vi "RTG_QMH_Main.vi"() -> ()   [LabVIEW 2020]
uses:
  <vilib>/RTG/API/interface/public/State.ctl
  <vilib>/RTG/API/ip/common/host-types/Target Configuration.ctl
  <vilib>/RTG/API/ip/common/host-types/Synchronization - Host.ctl
  <vilib>/RTG/API/ip/common/host-types/Synchronization Mode - Host.ctl
  <vilib>/RTG/API/ip/common/host-types/Basic Target - Host.ctl
  <vilib>/RTG/API/ip/common/host-types/Target Motion Parameters.ctl
  <vilib>/RTG/API/ip/common/host-types/Single Target Motion Parameters.ctl
  <vilib>/RTG/API/interface/public/Coprocessor Link Status.ctl
  <vilib>/RTG/coprocessor/host/RTG Coprocessor Link Interface/Public/Coprocessor Status.ctl
  Controls/Enum/Program_Status_Enum.ctl
  Controls/Enum/Supervisor_Enum.ctl
  Controls/Enum/RTG_Enum.ctl
  Controls/Clust/RTG Clust.ctl
  <vilib>/RTG/API/interface/NI-RTG Interface.lvclass
  Controls/Clust/CoProcessor Clust.ctl
  <vilib>/RTG/coprocessor/host/RTG Coprocessor Link Interface/RTG Coprocessor Link Interface.lvclass
  Controls/Enum/CoProcessor_Enum.ctl
  Controls/Clust/RTG API Clust.ctl
  support/Options - API Mode.ctl
  support/Options - Calibration.ctl
  support/Options - Remote.ctl
  <vilib>/Utility/error.llb/Error Cluster From Error Code.vi
  <vilib>/rvi/errors/niLvFpgaAdjustHostInterfaceError.vi
  <vilib>/rvi/interface/nirviReadWriteControl/nirviReadWriteControl.xnode
  RTG Examples.lvlib
  <vilib>/RTG/API/ip/common/host-types/Host Data Types v1.lvlib
  NiFpgaLv.dll
  <vilib>/rvi/interface/Simulation/niFpgaSimulationCallBeginRW.vi
panel:
  out "App Status":T1
  in  "Tab Control":T2(tab)
  in  "Instrument Names":string[](array[string])=["5831_0"]
  in  "Coprocessor Names":string[](array[string])
  in  "Center Freqeuncies (Hz)":dbl[](array[numeric])=[5500000000.0] format="%#_6p"
  in  "Reference Levels (dBm)":dbl[](array[numeric])=[0.0]
  in  "Calibrate":bool=TRUE
  in  "abort system self cal":bool
  in  "Commit HW":bool
  in  "ExtAtten":dbl[](array[numeric]) caption="External Attenuations (dB)"
  in  "OffsFreq":dbl[](array[numeric]) caption="Offset Frequencies (Hz)" format="%#_6p"
  in  "ExtDelay":dbl[](array[numeric]) caption="External Delay (s)" format="%#_6p"
  in  "mmWave Radio Heads Enable":bool[](array[boolean])
  in  "PRI (s)":dbl[](array[numeric]) format="%#_6p"
  in  "Set PRIs":bool
  out "Min Latencies (s)":dbl[](array[numeric]) format="%#_6p"
  out "Min Common Attenuations (dB)":dbl[](array[numeric])
  out "Max Common Attenuations (dB)":dbl[](array[numeric])
  out "Versions":string[](array[string])
  in  "Common Attenuation (dB)":dbl
  in  "Auto Send Software Trigger":bool
  in  "Prepend Software Trigger":bool
  in  "Device Index":i32
  in  "Target Configuration Files":path[](array[path])
  in  "Target Configuration":T3 {"rtg targets"."time offset (s)" format="%#_6p"; "rtg targets"."doppler" format="%#_6p"}
  in  "Target Motion Parameters":T7={"target motions"=[{"target enable"=FALSE, "start time offset (s)"=-1e-09, "time offset rate of change (s/s)"=0.001, "start attenuation (dB)"=0.0, "attenuation rate of change (dB/s)"=0.0, "start frequency shift (Hz)"=0.0, "frequency shift rate of change (Hz/sec)"=0.0}], "scenario duration (s)"=67.0, "configuration update rate(Hz)"=15000.0} {"configuration update rate(Hz)" format="%#_6p"; "target motions"."frequency shift rate of change (Hz/sec)" format="%#_6p"; "target motions"."start frequency shift (Hz)" format="%#_6p"; "target motions"."time offset rate of change (s/s)" format="%#_6p"; "target motions"."start time offset (s)" format="%#_6p"}
  in  "Send TrgtCfg":bool
  in  "Send Motion":bool
  in  "Send Files":bool
  in  "Start RTG":bool
  in  "Stop RTG":bool
  in  "Send SW Trigg":bool
  out "rtg link status":T9[](array[typedef])
  out "Trigger Count":i32[][](array[numeric]) caption="Device Index vs Trigger Count"
  out "RTG Status":string
  out "RTG State":T10
  out "error out":errorcluster
  out "System Time":string
  out "coproc link":T11[](array[typedef]) caption="coprocessor link status"
  in  "Exit":bool
  # "v20230906"
  # "Configuration Files and Target Motion"
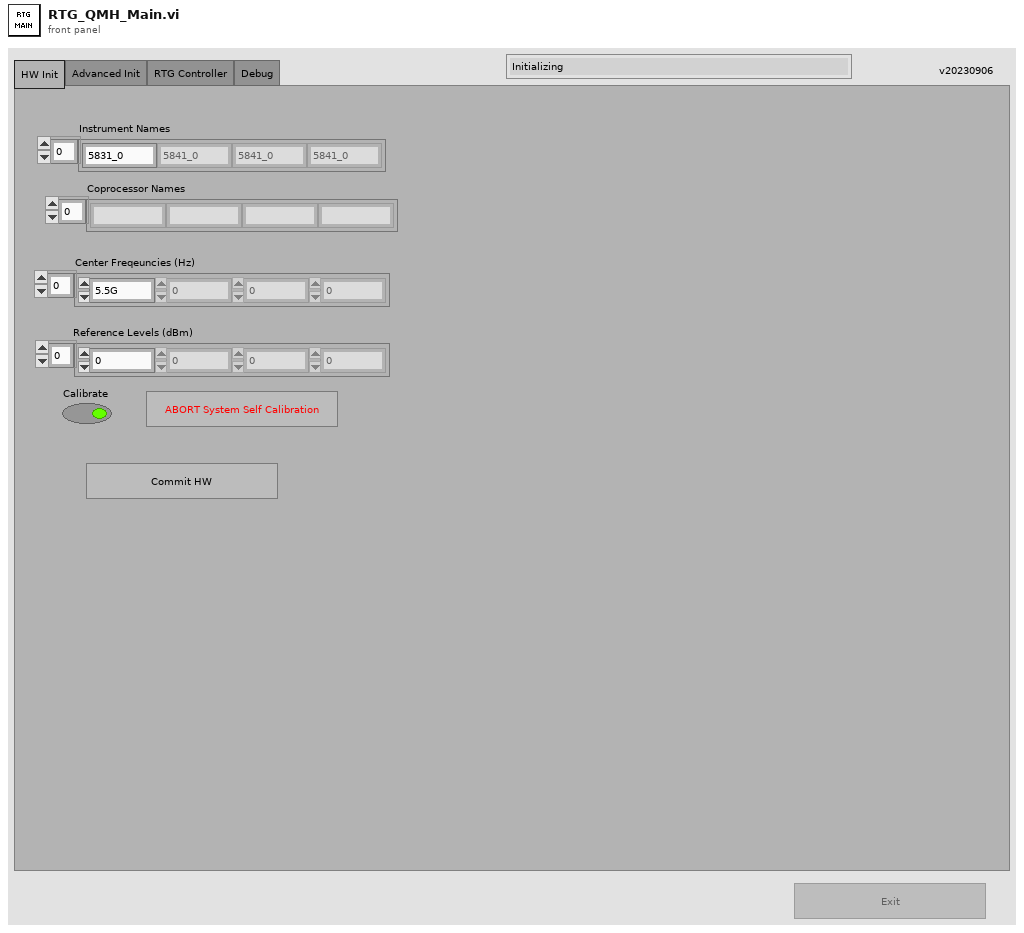
[diagram p1: front panel]
types:
  T1 = typedef "Program_Status_Enum.ctl" = enum16{"Initializing", "RTG Inactive", "Unconfigured", "RTG active", "Error", "Closing", "Closed"}
  T2 = enum32{"HW Init", "Advanced Init", "RTG Controller", "Debug"}
  T3 = typedef "Host Data Types v1.lvlib/Target Configuration.ctl" = cluster{"synchronization":T4, "rtg targets":T6[]}
  T4 = typedef "Host Data Types v1.lvlib/Synchronization - Host.ctl" = cluster{"synch mode":T5, "time offset (s)":dbl}
  T5 = typedef "Host Data Types v1.lvlib/Synchronization Mode - Host.ctl" = enum16{"Software Trigger", "Hardware Trigger", "Time Offset Relative to First", "Time Offset Relative to Last", "Pulse Rising Edge", "Pulse Falling Edge"}
  T6 = typedef "Host Data Types v1.lvlib/Basic Target - Host.ctl" = cluster{"time offset (s)":dbl, "attenuaton (dB)":dbl, "doppler":dbl, "target enable":bool, "relative velocity enable":bool}
  T7 = typedef "Host Data Types v1.lvlib/Target Motion Parameters.ctl" = cluster{"target motions":T8[], "scenario duration (s)":dbl, "configuration update rate(Hz)":dbl}
  T8 = typedef "Host Data Types v1.lvlib/Single Target Motion Parameters.ctl" = cluster{"target enable":bool, "start time offset (s)":dbl, "time offset rate of change (s/s)":dbl, "start attenuation (dB)":dbl, "attenuation rate of change (dB/s)":dbl, "start frequency shift (Hz)":dbl, "frequency shift rate of change (Hz/sec)":dbl}
  T9 = typedef "NI-RTG v1.lvlib/NI-RTG Interface.lvclass/Coprocessor Link Status.ctl" = cluster{"task name":string, "device name":string, "hard error":bool, "soft error":bool, "channel up":bool, "system reset":bool}
  T10 = typedef "NI-RTG v1.lvlib/NI-RTG Interface.lvclass/State.ctl" = enum16{"Idle", "Inactive", "Active", "System Self Calibration"}
  T11 = typedef "RTG Coprocessor Link Interface v1 Host.lvlib/RTG Coprocessor Link Interface.lvclass/Coprocessor Status.ctl" = cluster{"tx read count":u64, "tx read overflow":bool, "rx read count":u64, "rx read overflow":bool}
  T12 = typedef "CoProcessor_Enum.ctl" = enum16{"CoPr_Init", "CoPr_Chk", "CoPr_Exit"}
  T13 = typedef "CoProcessor Clust.ctl" = cluster{"CoPr Refs":refnum<class "RTG Coprocessor Link Interface.lvclass">[]}
  T14 = typedef "RTG Clust.ctl" = cluster{"VST_Names":string[], "OptionString":string, "RTG Ref":refnum<class "NI-RTG Interface.lvclass">, "Index":i32, "AutoSend":bool, "Prepend":bool, "state":T10}
  T15 = typedef "RTG_Enum.ctl" = enum16{"RTG_InitHW", "RTG_RefLvl", "RTG_mmWav", "RTG_Cal", "RTG_CalDone?", "RTG_ExtAtten", "RTG_GetCal", "RTG_SetPRIs", "RTG_CommAtten", "RTG_TargetSetup", "RTG_Send Files", "RTG_Send Target Cfg", "RTG_Send Motion", "RTG_Send SW Trigg", "RTG_Start", "RTG_Stop", "RTG_Chk", "RTG_Exit"}
  T16 = typedef "Supervisor_Enum.ctl" = enum16{"Spvsr_InitSW", "Spvsr_InitCtrls", "Spvsr_UpdtFP", "Spvsr_InitRTG", "Spvsr_StateCount", "Spvsr_Exit"}
  T17 = enum8{"Enabled", "Disabled", "Disabled and Grayed Out"}
  T18 = typedef "RTG API Clust.ctl" = cluster{"Local?":T19, "Cal":T20, "Remote":T21, "ini path":path}
  T19 = typedef "RTG Examples.lvlib/Options - API Mode.ctl" = enum16{"Local", "Remote"}
  T20 = typedef "RTG Examples.lvlib/Options - Calibration.ctl" = cluster{"enable internal loopback  ":bool, "enable overwrite cal data  ":bool, "enable save cal data           ":bool, "disable self cal range          ":bool}
  T21 = typedef "RTG Examples.lvlib/Options - Remote.ctl" = cluster{"ip address":string, "port":string, "certificate path":path, "timeout (ms)":i32}
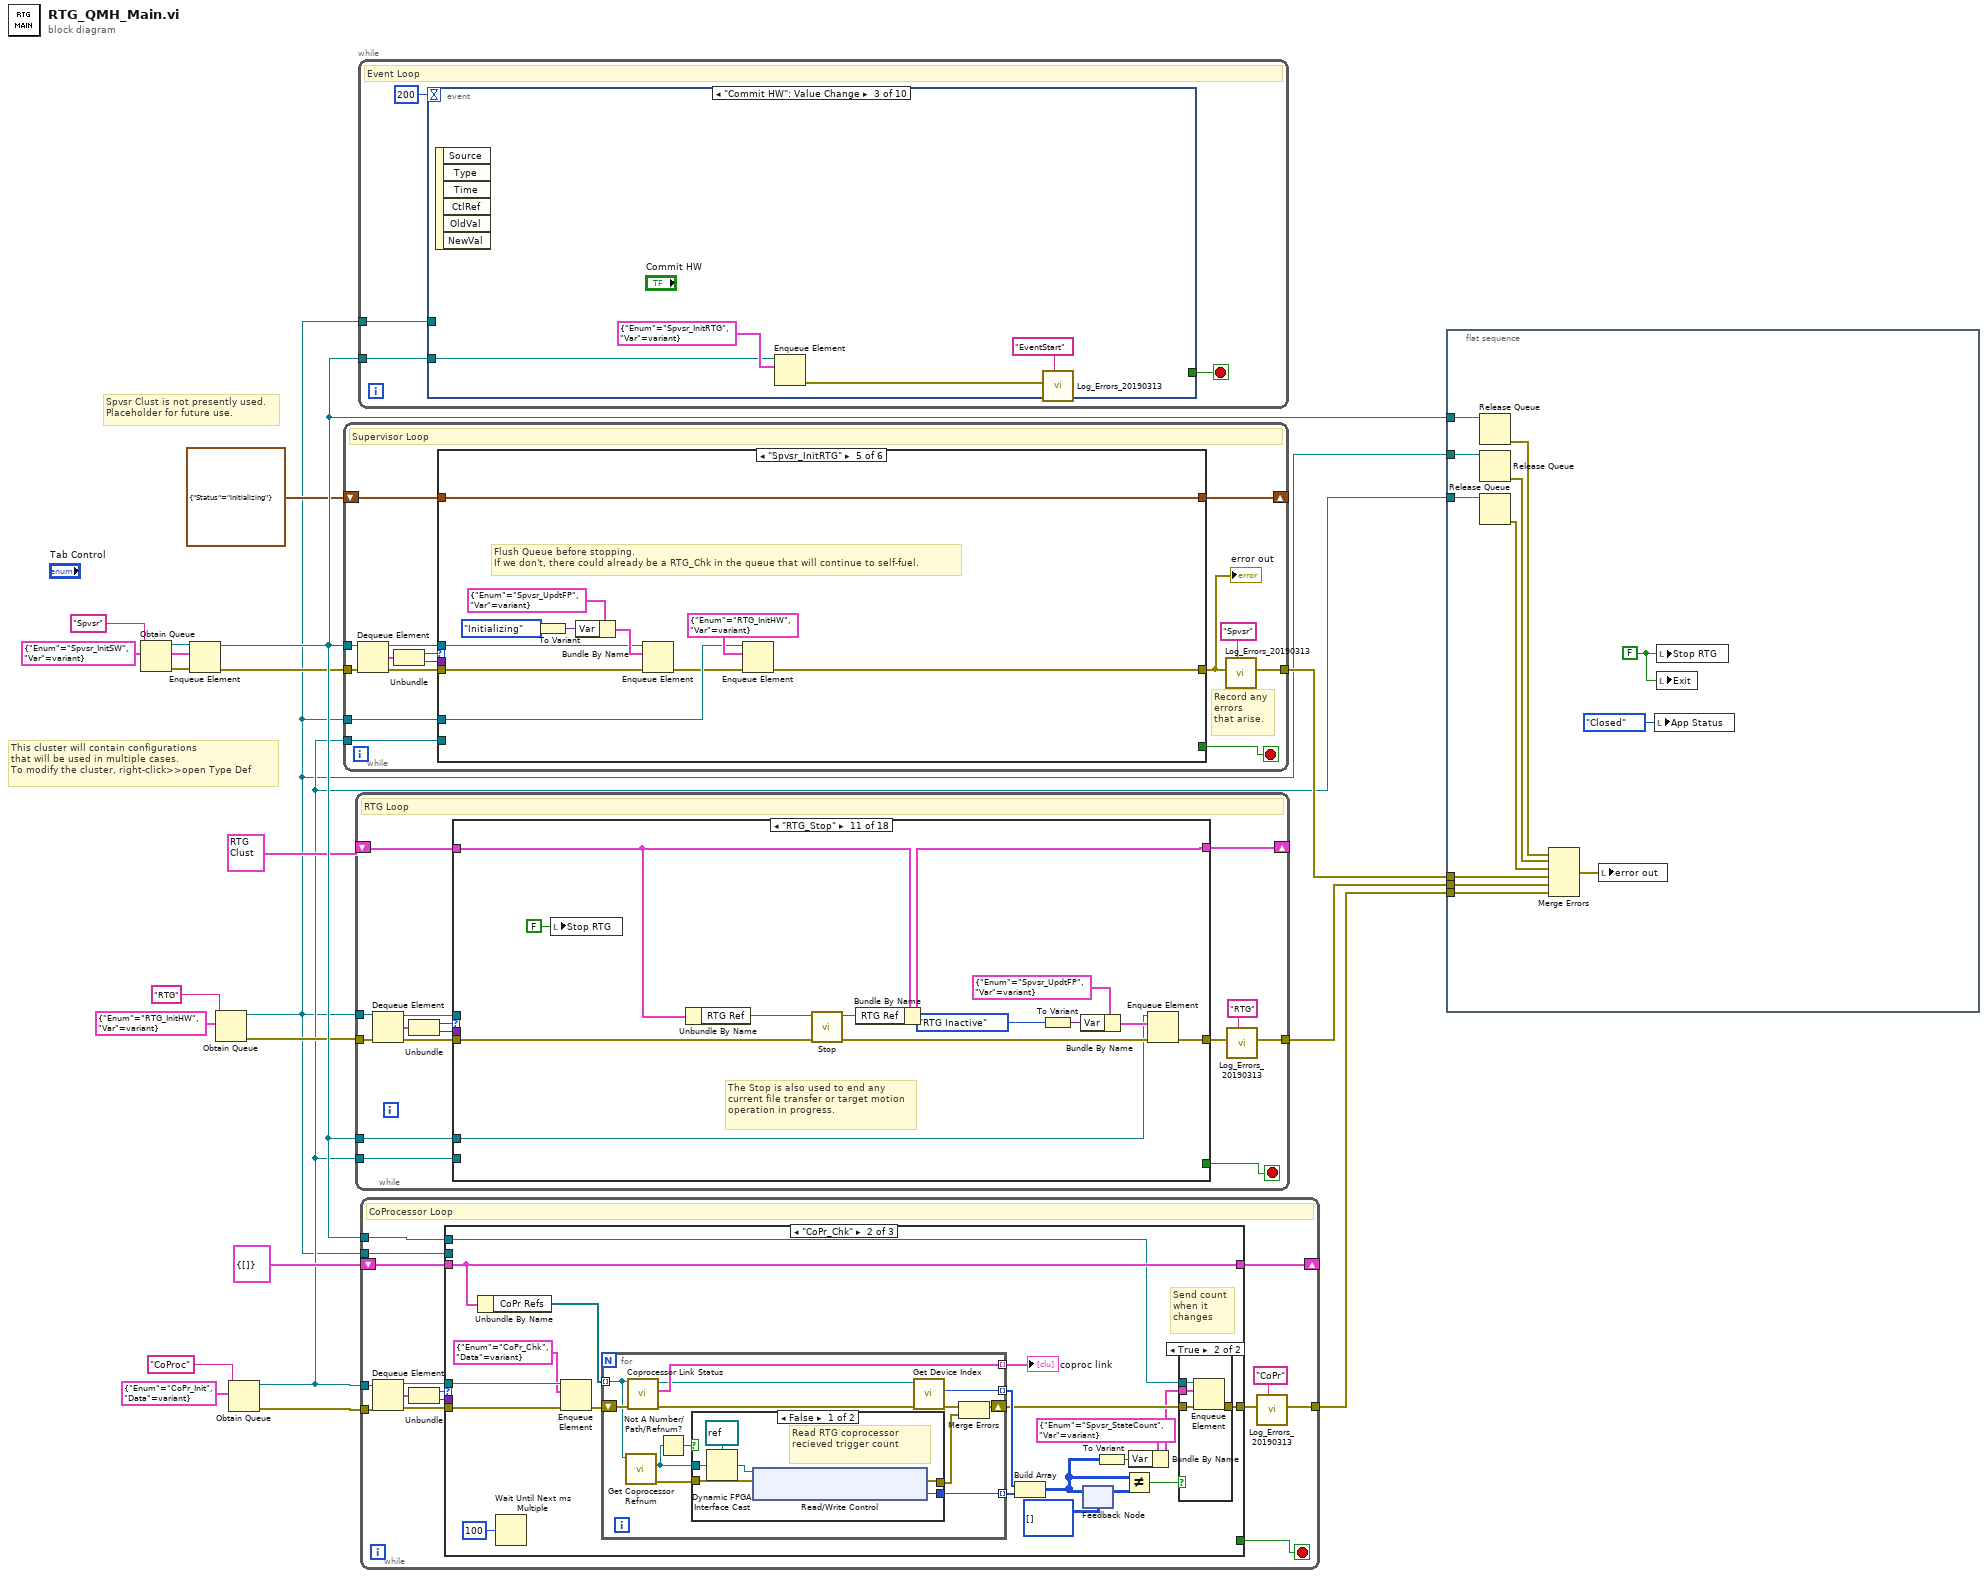
[diagram p0: block diagram]
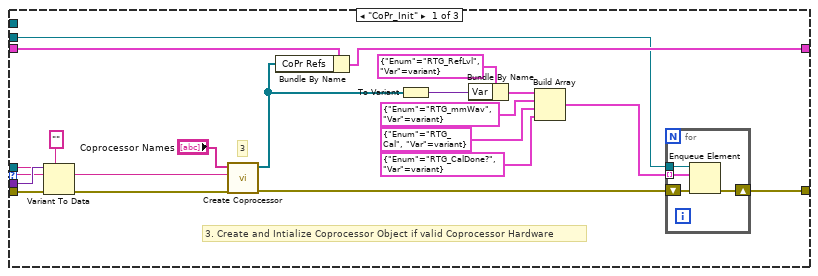
[diagram p2: hidden frame]
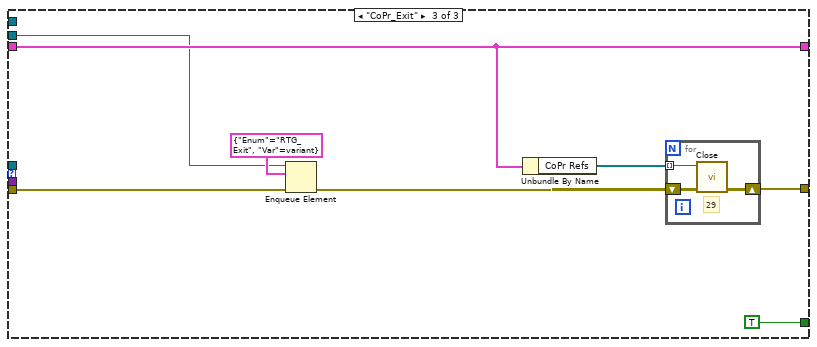
[diagram p5: hidden frame]
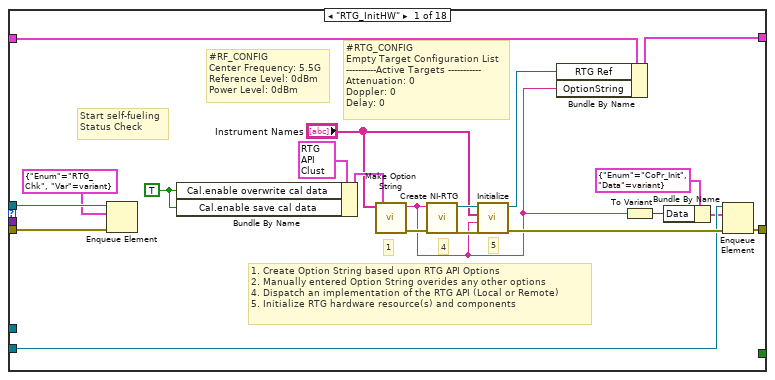
[diagram p6: hidden frame]
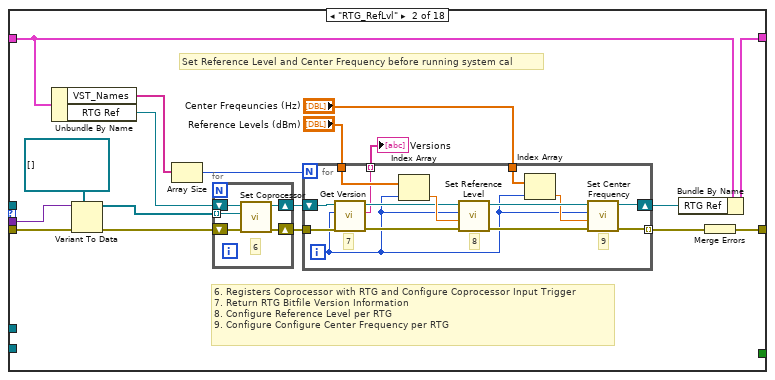
[diagram p7: hidden frame]
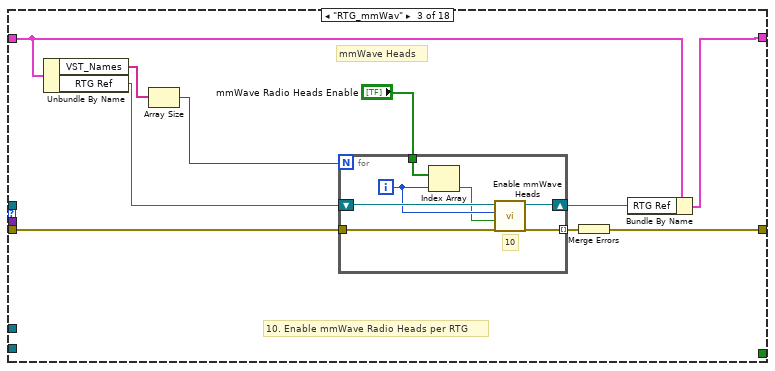
[diagram p8: hidden frame]
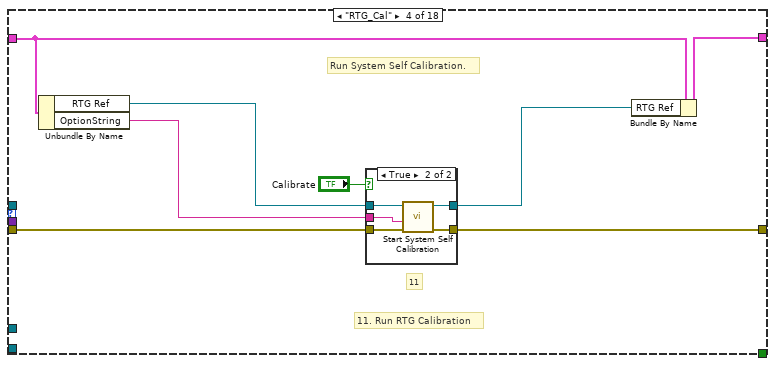
[diagram p9: hidden frame]
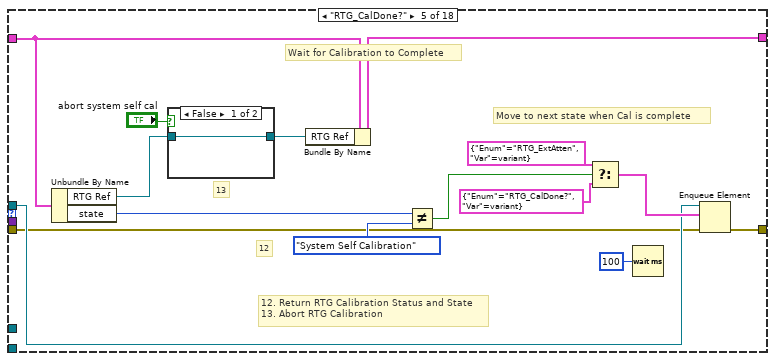
[diagram p11: hidden frame]
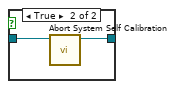
[diagram p12: hidden frame]
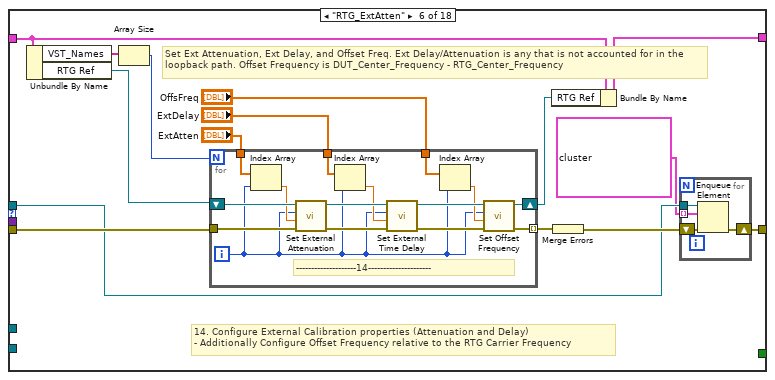
[diagram p13: hidden frame]
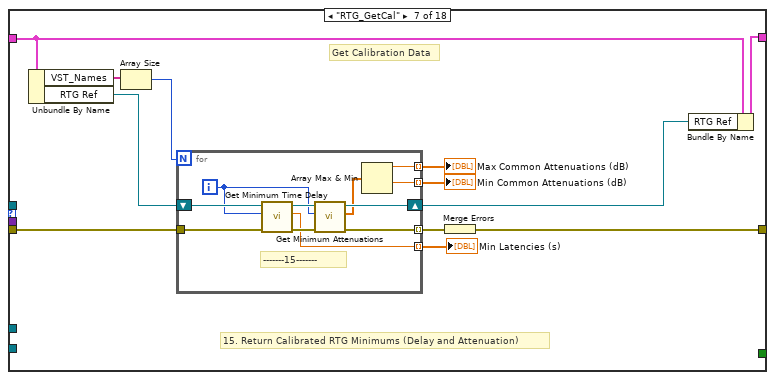
[diagram p14: hidden frame]
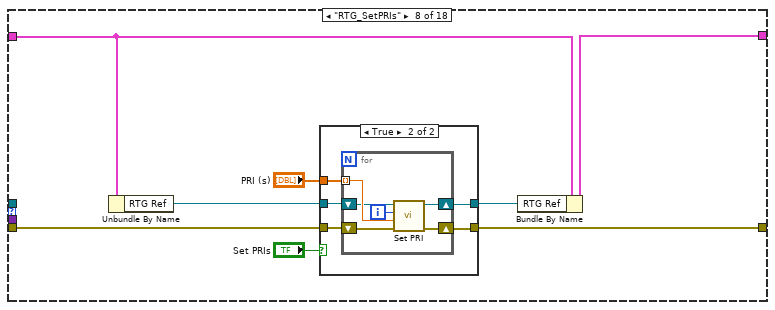
[diagram p15: hidden frame]
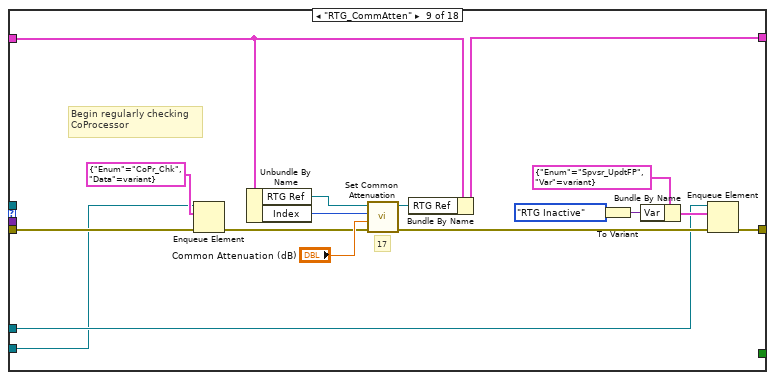
[diagram p17: hidden frame]
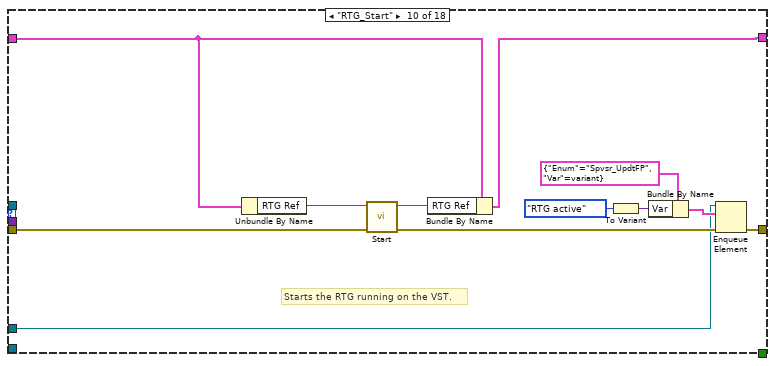
[diagram p18: hidden frame]
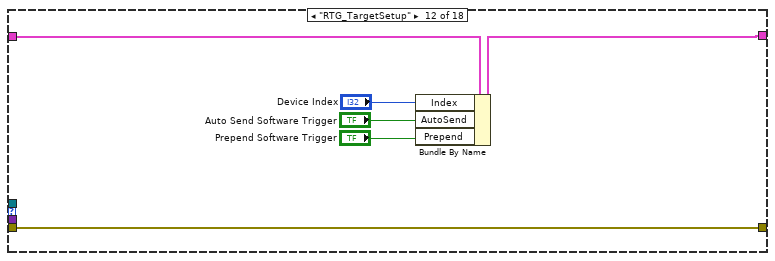
[diagram p19: hidden frame]
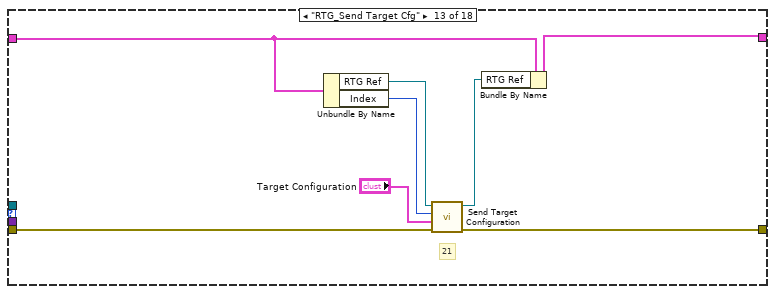
[diagram p20: hidden frame]
diagram:
  w16 = cluster{"Enum":T16, "Var":variant} {"Enum"=enum."Spvsr_InitSW", "Var"=variant}
  # "Spvsr Clust is not presently used.\nPlaceholder for future use."
  # "This cluster will contain configurations\nthat will be used in multiple cases.\nTo modify the cluster, right-click>>open Type Def"
  n1 = Obtain Queue(name (unnamed)="Spvsr", element data type=w16) -> (queue out=w17:refnum<queue>, error out=w19:errorcluster)  [unwired: 3 in, 1 out]
  n2 = Enqueue Element(queue=w17, element=w16, error in (no error)=w19) -> (queue out=w20:refnum<queue>, error out=w18:errorcluster)  [unwired: 1 in, 1 out]
  n3 = Obtain Queue(name (unnamed)="RTG", element data type=cluster{"Enum":T15, "Var":variant} {"Enum"=enum."RTG_InitHW", "Var"=variant}) -> (queue out=w1:refnum<queue>, error out=w14:errorcluster)  [unwired: 3 in, 1 out]
  n4 = Obtain Queue(name (unnamed)="CoProc", element data type=cluster{"Enum":T12, "Data":variant} {"Enum"=enum."CoPr_Init", "Data"=variant}) -> (queue out=w2:refnum<queue>, error out=w12:errorcluster)  [unwired: 3 in, 1 out]
  n5 = while {
    tunnel: w18 -> [w35]
    tunnel: w20 -> [w33]
    tunnel: w1 -> [w28]
    tunnel: [w25] -> w6
    tunnel: w2 -> [w24]
    shift-right: [w22] -> _
    shift-left: cluster{"Status":T1} {"Status"=enum."Initializing"} -> [w23]
    stop <- w21 stop-if-true
    # "Record any\nerrors \nthat arise."
    # "Supervisor Loop"
    n6 = Dequeue Element(queue=w33, error in (no error)=w35) -> (queue out=w31:refnum<queue>, element=w32:cluster{"Enum":T16, "Var":variant}, error out=w34:errorcluster)  [unwired: 1 in, 1 out]
    n7 = Unbundle(w32) -> ("Enum"=w30:T16, "Var"=w29:variant)
    n8 = case shown="\"Spvsr_InitRTG\"" w30 {
      tunnel: w34 -> [w46 w48 w59 w121 w127 w139]
      tunnel: w31 -> [w45 w47 _ _ w124 _]
      tunnel: w29 -> [_ _ w58 _ _ w137]
      tunnel: w28 -> [_ _ _ w119 w133 _]
      tunnel: [w43 w49 w61 w118 w125 w135] -> w26
      tunnel: w24 -> [_ _ _ w116 _ _]
      tunnel: w23 -> [w36 w54 w74 w112 w132 w140]
      tunnel: [w36 w54 w74 w112 w132 w140] -> w22
      tunnel: [_ _ _ TRUE _ _] -> w21
      frame "Spvsr_InitSW" {
        n9 = Enqueue Element(queue=w45, element=cluster{"Enum":T16, "Var":variant} {"Enum"=enum."Spvsr_InitCtrls", "Var"=variant}, error in (no error)=w46) -> (queue out=w41:refnum<queue>, error out=w42:errorcluster)  [unwired: 1 in, 1 out]
        n10 = To Variant(anything=Program_Status_Enum."Initializing" ("Status")) -> (Variant=w38:variant)
        n11 = Bundle By Name(cluster=cluster{"Enum":T16, "Var":variant} {"Enum"=enum."Spvsr_UpdtFP", "Var"=variant}, "Var"=w38) -> (w37:cluster{"Enum":T16, "Var":variant})
        n12 = Enqueue Element(queue=w41, element=w37, error in (no error)=w42) -> (error out=w43:errorcluster)  [unwired: 1 in, 2 out]
      }
      frame "Spvsr_InitCtrls" {
        w55 = FALSE ("Exit")
        n13 = To Variant(anything=Program_Status_Enum."Unconfigured" ("Status")) -> (Variant=w53:variant)
        n14 = Bundle By Name(cluster=cluster{"Enum":T16, "Var":variant} {"Enum"=enum."Spvsr_UpdtFP", "Var"=variant}, "Var"=w53) -> (w51:cluster{"Enum":T16, "Var":variant})
        n15 = Enqueue Element(queue=w47, element=w51, error in (no error)=w48) -> (error out=w49:errorcluster)  [unwired: 1 in, 2 out]
        n16 = local write "Exit"(w55) -> ()
        n17 = local write "Stop RTG"(w55) -> ()
      }
      frame "Spvsr_UpdtFP" {
        n18 = Variant To Data(error in=w59, type=Program_Status_Enum."Closed" ("App Status"), Variant=w58) -> (data=w56:T1, error out=w60:errorcluster)
        "App Status" <- w56
        n19 = case shown="\"Unconfigured\"" w56 {
          tunnel: [T17."Disabled and Grayed Out" ("Disabled") T17."Enabled" ("Disabled") T17."Disabled and Grayed Out" ("Disabled") T17."Disabled and Grayed Out" ("Disabled") T17."Enabled" ("Disabled") T17."Disabled and Grayed Out" ("Disabled")] -> w67
          tunnel: [T17."Disabled and Grayed Out" ("Disabled") T17."Enabled" ("Disabled") T17."Disabled and Grayed Out" ("Disabled") T17."Disabled and Grayed Out" ("Disabled") T17."Disabled and Grayed Out" ("Disabled") T17."Enabled" ("Disabled")] -> w66
          tunnel: [T17."Enabled" ("Disabled") T17."Enabled" ("Disabled") T17."Disabled and Grayed Out" ("Disabled") T17."Enabled" ("Disabled") T17."Enabled" ("Disabled") T17."Enabled" ("Disabled")] -> w65
          tunnel: [T17."Disabled and Grayed Out" ("Disabled") T17."Disabled and Grayed Out" ("Disabled") T17."Disabled and Grayed Out" ("Disabled") T17."Disabled and Grayed Out" ("Disabled") T17."Disabled and Grayed Out" ("Disabled") T17."Enabled" ("Disabled")] -> w64
          tunnel: [T17."Disabled and Grayed Out" ("Disabled") T17."Disabled and Grayed Out" ("Disabled") T17."Disabled and Grayed Out" ("Disabled") T17."Disabled and Grayed Out" ("Disabled") T17."Disabled and Grayed Out" ("Disabled") T17."Enabled" ("Disabled")] -> w63
          tunnel: [T17."Disabled and Grayed Out" ("Disabled") T17."Disabled and Grayed Out" ("Disabled") T17."Disabled and Grayed Out" ("Disabled") T17."Disabled and Grayed Out" ("Disabled") T17."Disabled and Grayed Out" ("Disabled") T17."Enabled" ("Disabled")] -> w62
          frame "Unconfigured" {
          }
          frame "Error" {
          }
          frame "Closing", "Closed" {
          }
          frame "Initializing" {
          }
          frame "RTG Inactive" {
          }
          frame "RTG active" {
          }
        }
        n20 = property on="Start RTG" class="Bool"(error in=w60, "DisabledEnum"=w67) -> (error out=w68:errorcluster)  [unwired: 1 in, 1 out]
        n21 = property on="Stop RTG" class="Bool (strict)"("DisabledEnum"=w66) -> (error out=w69:errorcluster)  [unwired: 2 in, 1 out]
        n22 = property on="Exit" class="Bool (strict)"("DisabledEnum"=w65) -> (error out=w70:errorcluster)  [unwired: 2 in, 1 out]
        n23 = property on="Send TrgtCfg" class="Bool"("DisabledEnum"=w64) -> (error out=w71:errorcluster)  [unwired: 2 in, 1 out]
        n24 = property on="Send Motion" class="Bool"("DisabledEnum"=w63) -> (error out=w72:errorcluster)  [unwired: 2 in, 1 out]
        n25 = property on="Send Files" class="Bool"("DisabledEnum"=w62) -> (error out=w73:errorcluster)  [unwired: 2 in, 1 out]
        n26 = Merge Errors(w68, w69, w70, w71, w72, w73) -> (w61:errorcluster)
      }
      frame "Spvsr_Exit" {
        # "RTG Exit is called from Coprocesor Exit\nto prevent a race condition"
        # "Flush Queue before stopping.\nIf we don't, there could already be a RTG_Chk in the queue that will continue to self-fuel."
        n27 = Flush Queue(queue=w119, error in (no error)=w121) -> (queue out=w120:refnum<queue>, error out=w122:errorcluster)  [unwired: 1 out]
        n28 = Enqueue Element(queue=w120, element=cluster{"Enum":T15, "Var":variant} {"Enum"=enum."RTG_Stop", "Var"=variant}, error in (no error)=w122) -> (error out=w114:errorcluster)  [unwired: 1 in, 2 out]
        n29 = Flush Queue(queue=w116, error in (no error)=w114) -> (queue out=w115:refnum<queue>, error out=w113:errorcluster)  [unwired: 1 out]
        n30 = Enqueue Element(queue=w115, element=cluster{"Enum":T12, "Data":variant} {"Enum"=enum."CoPr_Exit", "Data"=variant}, error in (no error)=w113) -> (error out=w118:errorcluster)  [unwired: 1 in, 2 out]
      }
      frame "Spvsr_InitRTG" {
        # "Flush Queue before stopping.\nIf we don't, there could already be a RTG_Chk in the queue that will continue to self-fuel."
        n31 = To Variant(anything=Program_Status_Enum."Initializing" ("Status")) -> (Variant=w131:variant)
        n32 = Bundle By Name(cluster=cluster{"Enum":T16, "Var":variant} {"Enum"=enum."Spvsr_UpdtFP", "Var"=variant}, "Var"=w131) -> (w129:cluster{"Enum":T16, "Var":variant})
        n33 = Enqueue Element(queue=w124, element=w129, error in (no error)=w127) -> (error out=w126:errorcluster)  [unwired: 1 in, 2 out]
        n34 = Enqueue Element(queue=w133, element=cluster{"Enum":T15, "Var":variant} {"Enum"=enum."RTG_InitHW", "Var"=variant}, error in (no error)=w126) -> (error out=w125:errorcluster)  [unwired: 1 in, 2 out]
      }
      frame "Spvsr_StateCount" {
        # "Making this value available to the rest of the program."
        n35 = Variant To Data(error in=w139, type=i32[][] [] ("appended array"), Variant=w137) -> (data=→"Trigger Count":i32[][], error out=w135:errorcluster)
      }
    }
    "error out" <- w26
    n36 = call "Log_Errors_20190313.vi"("LoopName"="Spvsr", "error in"=w26) -> ("error out"=w25:errorcluster)  [unwired: 9 in]
  }
  n37 = while {
    tunnel: w14 -> [w155]
    shift-right: [w147] -> _
    shift-left: T14 {"VST_Names"=["5841_0"], "OptionString"="", "RTG Ref"=refnum, "Index"=0, "AutoSend"=FALSE, "Prepend"=FALSE, "state"=enum."Idle"} ("DAQ Clust") -> [w148]
    tunnel: [w145] -> w5
    tunnel: w2 -> [w144]
    tunnel: w1 -> [w142]
    tunnel: w20 -> [w141]
    stop <- w143 stop-if-true
    # "RTG Loop"
    n38 = Dequeue Element(queue=w142, error in (no error)=w155) -> (queue out=w152:refnum<queue>, element=w153:cluster{"Enum":T15, "Var":variant}, error out=w154:errorcluster)  [unwired: 1 in, 1 out]
    n39 = Unbundle(w153) -> ("Enum"=w151:T15, "Var"=w150:variant)
    n40 = case shown="\"RTG_Stop\"" w151 {
      tunnel: w154 -> [w158 w184 w217 w234 w246 w272 w301 w323 w342 w369 w378 w388 w395 w403 w432 w459 w471 w481]
      tunnel: w152 -> [w157 _ _ _ w249 w264 _ _ _ _ _ _ _ _ _ _ w470 _]
      tunnel: w150 -> [_ w181 _ _ _ _ _ _ _ _ _ _ _ _ _ _ _ _]
      tunnel: w148 -> [w175 w178 w213 w237 w259 w277 w307 w327 w357 w365 w381 w386 w392 w410 w439 w461 w476 w478]
      tunnel: [w174 w177 w214 w236 w258 w276 w308 w326 w356 w366 w382 w387 w391 w409 w438 w460 w475 w478] -> w147
      tunnel: [w164 w179 w216 w233 w248 w265 w300 w322 w348 w359 w371 w388 w394 w402 w431 w458 w465 w480] -> w146
      tunnel: w144 -> [w163 _ _ _ _ _ _ _ w341 _ _ _ _ _ _ _ _ _]
      tunnel: [_ _ _ _ _ _ _ _ _ _ _ _ _ _ _ _ _ TRUE] -> w143
      tunnel: w141 -> [_ _ _ _ _ _ _ _ w345 w358 w370 _ _ _ _ _ _ _]
      frame "RTG_InitHW" {
        w173 = TRUE ("Calibration Options.enable overwrite cal data")
        # "Start self-fueling\nStatus Check"
        # "1. Create Option String based upon RTG API Options\n2. Manually entered Option String overides any other options\n4. Dispatch an implementation of the RTG API (Local or Remote)\n5. Initialize RTG hardware resource(s) and components"
        # "#RTG_CONFIG\nEmpty Target Configuration List\n----------Active Targets -----------\nAttenuation: 0\nDoppler: 0\nDelay: 0"
        # "#RF_CONFIG\nCenter Frequency: 5.5G\nReference Level: 0dBm\nPower Level: 0dBm"
        # "4"
        # "1"
        # "5"
        n41 = Enqueue Element(queue=w157, element=cluster{"Enum":T15, "Var":variant} {"Enum"=enum."RTG_Chk", "Var"=variant}, error in (no error)=w158) -> ()  [unwired: 1 in, 3 out]
        n42 = Bundle By Name(cluster=T18 {"Local?"=enum."Local", "Cal"={"enable internal loopback  "=FALSE, "enable overwrite cal data  "=FALSE, "enable save cal data           "=FALSE, "disable self cal range          "=FALSE}, "Remote"={"ip address"="", "port"="50052", "certificate path"=path "", "timeout (ms)"=15000}, "ini path"=path ""} ("RTG API Options"), "Cal.enable overwrite cal data"=w173, "Cal.enable save cal data"=w173) -> (w172:T18)
        n43 = call "Make Option String.vi"("RTG API Options"=w172, "instrument names"="Instrument Names") -> ("error out"=w171:errorcluster, "option string"=w161:string)  [unwired: 8 in]
        n44 = call <vilib>:"Create NI-RTG.vi"("error in"=w171, "option string"=w161) -> ("error out"=w169:errorcluster, "NI-RTG Interface out"=w168:refnum<class "NI-RTG Interface.lvclass">)  [unwired: 8 in]
        n45 = call-dynamic "Initialize.vi"("error in"=w169, "option string"=w161, "instrument names"="Instrument Names", "ni-rtg interface"=w168) -> ("error out"=w165:errorcluster, "ni-rtg interface out"=w166:refnum<class "NI-RTG Interface.lvclass">)  [unwired: 6 in]
        n46 = Bundle By Name(cluster=w175, "RTG Ref"=w166, "OptionString"=w161) -> (w174:T14)
        n47 = To Variant(anything=w161) -> (Variant=w160:variant)
        n48 = Bundle By Name(cluster=cluster{"Enum":T12, "Data":variant} {"Enum"=enum."CoPr_Init", "Data"=variant}, "Data"=w160) -> (w159:cluster{"Enum":T12, "Data":variant})
        n49 = Enqueue Element(queue=w163, element=w159, error in (no error)=w165) -> (error out=w164:errorcluster)  [unwired: 1 in, 2 out]
      }
      frame "RTG_RefLvl" {
        # "6. Registers Coprocessor with RTG and Configure Coprocessor Input Trigger\n7. Return RTG Bitfile Version Information\n8. Configure Reference Level per RTG\n9. Configure Configure Center Frequency per RTG"
        # "Set Reference Level and Center Frequency before running system cal"
        n50 = Unbundle By Name(w178) -> ("VST_Names"=w186:string[], "RTG Ref"=w187:refnum<class "NI-RTG Interface.lvclass">)
        n51 = Variant To Data(error in=w184, type=refnum<class "RTG Coprocessor Link Interface.lvclass">[] [] ("rtg coprocessor links"), Variant=w181) -> (data=w180:refnum<class "RTG Coprocessor Link Interface.lvclass">[], error out=w183:errorcluster)
        n52 = Array Size(array=w186) -> (size(s)=w185:i32)
        n53 = for {
          shift-right: [w212] -> w191
          shift-left: w183 -> [w210]
          shift-right: [w211] -> w192
          shift-left: w187 -> [w209]
          tunnel: w180 -> [w208] mode=indexing
          # "6"
          n54 = call-dynamic "Set Coprocessor.vi"("error in"=w210, "rtg coprocessor link interface"=w208, "rtg api interface"=w209) -> ("error out"=w212:errorcluster, "rtg api interface out"=w211:refnum<class "NI-RTG Interface.lvclass">)  [unwired: 7 in]
        }
        n55 = for {
          N: w185 -> [_]
          tunnel: w191 -> [w197]
          tunnel: "Reference Levels (dBm)" -> [w205]
          tunnel: "Center Freqeuncies (Hz)" -> [w203]
          shift-right: [w201] -> w176
          shift-left: w192 -> [w199]
          tunnel: [w200] -> w190 mode=indexing
          tunnel: [w194] -> w193 mode=indexing
          i -> [w195]
          # "9"
          # "8"
          # "7"
          n56 = call-dynamic "Get Version.vi"("error in"=w197, "device index (0)"=w195, "NI-RTG Interface in"=w199) -> ("error out"=w196:errorcluster, "version"=w194:string, "NI-RTG Interface out"=w198:refnum<class "NI-RTG Interface.lvclass">)  [unwired: 6 in]
          n57 = Index Array(array=w205, index=w195) -> (element=w204:dbl)
          n58 = call-dynamic "Set Reference Level.vi"("error in"=w196, "reference level (dBm)"=w204, "device index (0)"=w195, "rtg api interface"=w198) -> ("error out"=w206:errorcluster, "rtg api interface out"=w207:refnum<class "NI-RTG Interface.lvclass">)  [unwired: 6 in]
          n59 = Index Array(array=w203, index=w195) -> (element=w202:dbl)
          n60 = call-dynamic "Set Center Frequency.vi"("error in"=w206, "center frequency (Hz)"=w202, "device index (0)"=w195, "rtg api interface"=w207) -> ("error out"=w200:errorcluster, "rtg api interface out"=w201:refnum<class "NI-RTG Interface.lvclass">)  [unwired: 6 in]
        }
        "Versions" <- w193
        n61 = Bundle By Name(cluster=w178, "RTG Ref"=w176) -> (w177:T14)
        n62 = Merge Errors(w190) -> (w179:errorcluster)
      }
      frame "RTG_mmWav" {
        # "10. Enable mmWave Radio Heads per RTG"
        # "mmWave Heads"
        n63 = Unbundle By Name(w213) -> ("VST_Names"=w222:string[], "RTG Ref"=w219:refnum<class "NI-RTG Interface.lvclass">)
        n64 = Array Size(array=w222) -> (size(s)=w218:i32)
        n65 = for {
          N: w218 -> [_]
          shift-right: [w226] -> w215
          shift-left: w219 -> [w227]
          tunnel: w217 -> [w229]
          tunnel: [w228] -> w220 mode=indexing
          tunnel: "mmWave Radio Heads Enable" -> [w225]
          i -> [w224]
          # "10"
          n66 = Index Array(array=w225, index=w224) -> (element=w223:bool)
          n67 = call-dynamic "Enable mmWave Heads.vi"("error in"=w229, "enable mmWave"=w223, "device index (0)"=w224, "ni-rtg interface"=w227) -> ("error out"=w228:errorcluster, "ni-rtg interface out"=w226:refnum<class "NI-RTG Interface.lvclass">)  [unwired: 6 in]
        }
        n68 = Merge Errors(w220) -> (w216:errorcluster)
        n69 = Bundle By Name(cluster=w213, "RTG Ref"=w215) -> (w214:T14)
      }
      frame "RTG_Cal" {
        # "11"
        # "11. Run RTG Calibration"
        # "Run System Self Calibration."
        n70 = Unbundle By Name(w237) -> ("RTG Ref"=w232:refnum<class "NI-RTG Interface.lvclass">, "OptionString"=w230:string)
        n71 = case shown="True" "Calibrate" {
          tunnel: w232 -> [w239 w244]
          tunnel: w234 -> [w238 w243]
          tunnel: [w239 w242] -> w231
          tunnel: [w238 w241] -> w233
          tunnel: w230 -> [_ w240]
          frame False {
          }
          frame True {
            n72 = call-dynamic "Start System Self Calibration.vi"("error in"=w243, "option string"=w240, "rtg api interface"=w244) -> ("error out"=w241:errorcluster, "rtg api interface out"=w242:refnum<class "NI-RTG Interface.lvclass">)  [unwired: 7 in]
          }
        }
        n73 = Bundle By Name(cluster=w237, "RTG Ref"=w231) -> (w236:T14)
      }
      frame "RTG_CalDone?" {
        # "Move to next state when Cal is complete"
        # "13"
        # "12"
        # "12. Return RTG Calibration Status and State\n13. Abort RTG Calibration"
        # "Wait for Calibration to Complete"
        n74 = Unbundle By Name(w259) -> ("RTG Ref"=w257:refnum<class "NI-RTG Interface.lvclass">, "state"=w245:T10)
        n75 = case shown="False" "abort system self cal" {
          tunnel: w257 -> [w260 w262]
          tunnel: [w260 w261] -> w247
          frame False {
          }
          frame True {
            n76 = call-dynamic "Abort System Self Calibration.vi"("rtg-api interface"=w262) -> ("rtg-api interface out"=w261:refnum<class "NI-RTG Interface.lvclass">)  [unwired: 9 in, 1 out]
          }
        }
        n77 = Bundle By Name(cluster=w259, "RTG Ref"=w247) -> (w258:T14)
        n78 = Not Equal?(x=w245, y=State."System Self Calibration") -> (x != y?=w250:bool)
        n79 = Select(t=cluster{"Enum":T15, "Var":variant} {"Enum"=enum."RTG_ExtAtten", "Var"=variant} ("element"), s=w250, f=cluster{"Enum":T15, "Var":variant} {"Enum"=enum."RTG_CalDone?", "Var"=variant} ("element")) -> (s? t:f=w253:cluster{"Enum":T15, "Var":variant})
        n80 = Wait (ms)(milliseconds to wait=u32 100) -> ()  [unwired: 1 out]
        n81 = Enqueue Element(queue=w249, element=w253, error in (no error)=w246) -> (error out=w248:errorcluster)  [unwired: 1 in, 2 out]
      }
      frame "RTG_ExtAtten" {
        # "Set Ext Attenuation, Ext Delay, and Offset Freq. Ext Delay/Attenuation is any that is not accounted for in the loopback path. Offset Frequency is DUT_Center_Frequency - RTG_Center_Frequency"
        # "14. Configure External Calibration properties (Attenuation and Delay)\n- Additionally Configure Offset Frequency relative to the RTG Carrier Frequency"
        n82 = Unbundle By Name(w277) -> ("VST_Names"=w275:string[], "RTG Ref"=w268:refnum<class "NI-RTG Interface.lvclass">)
        n83 = Array Size(array=w275) -> (size(s)=w269:i32)
        n84 = for {
          N: w269 -> [_]
          shift-right: [w286] -> w267
          shift-left: w268 -> [w296]
          tunnel: "ExtAtten" -> [w294]
          tunnel: "ExtDelay" -> [w292]
          tunnel: [w288] -> w271 mode=indexing
          tunnel: w272 -> [w285]
          tunnel: "OffsFreq" -> [w284]
          i -> [w282]
          # "--------------------14---------------------"
          n85 = Index Array(array=w294, index=w282) -> (element=w293:dbl)
          n86 = call-dynamic "Set External Attenuation.vi"("error in"=w285, "external attenuation (dB)"=w293, "device index (0)"=w282, "rtg api interface"=w296) -> ("error out"=w290:errorcluster, "rtg api interface out"=w295:refnum<class "NI-RTG Interface.lvclass">)  [unwired: 6 in]
          n87 = Index Array(array=w292, index=w282) -> (element=w291:dbl)
          n88 = call-dynamic "Set External Time Delay.vi"("error in"=w290, "delay (s)"=w291, "device index (0)"=w282, "rtg api interface"=w295) -> ("error out"=w289:errorcluster, "rtg api interface out"=w287:refnum<class "NI-RTG Interface.lvclass">)  [unwired: 6 in]
          n89 = Index Array(array=w284, index=w282) -> (element=w283:dbl)
          n90 = call-dynamic "Set Offset Frequency.vi"("error in"=w289, "offset frequency (Hz)"=w283, "device index (0)"=w282, "NI-RTG Interface in"=w287) -> ("error out"=w288:errorcluster, "NI-RTG Interface out"=w286:refnum<class "NI-RTG Interface.lvclass">)  [unwired: 6 in]
        }
        n91 = Bundle By Name(cluster=w277, "RTG Ref"=w267) -> (w276:T14)
        n92 = Merge Errors(w271) -> (w266:errorcluster)
        n93 = for {
          tunnel: w264 -> [w279]
          tunnel: cluster{"Enum":T15, "Var":variant}[] [{"Enum"=enum."RTG_GetCal", "Var"=variant}, {"Enum"=enum."RTG_SetPRIs", "Var"=variant}, {"Enum"=enum."RTG_CommAtten", "Var"=variant}] -> [w278] mode=indexing
          shift-right: [w280] -> w265
          shift-left: w266 -> [w281]
          n94 = Enqueue Element(queue=w279, element=w278, error in (no error)=w281) -> (error out=w280:errorcluster)  [unwired: 1 in, 2 out]
        }
      }
      frame "RTG_GetCal" {
        # "15. Return Calibrated RTG Minimums (Delay and Attenuation)"
        # "Get Calibration Data"
        n95 = Unbundle By Name(w307) -> ("VST_Names"=w306:string[], "RTG Ref"=w298:refnum<class "NI-RTG Interface.lvclass">)
        n96 = Array Size(array=w306) -> (size(s)=w299:i32)
        n97 = for {
          N: w299 -> [_]
          tunnel: w301 -> [w319]
          tunnel: [w316] -> w302 mode=indexing
          shift-right: [w314] -> w297
          shift-left: w298 -> [w317]
          tunnel: [w313] -> w305 mode=indexing
          tunnel: [w311] -> w303 mode=indexing
          tunnel: [w310] -> w304 mode=indexing
          i -> [w309]
          # "-------15-------"
          n98 = call-dynamic "Get Minimum Time Delay.vi"("error in"=w319, "device index (0)"=w309, "rtg api interface"=w317) -> ("error out"=w318:errorcluster, "delay (s)"=w313:dbl, "rtg api interface out"=w315:refnum<class "NI-RTG Interface.lvclass">)  [unwired: 5 in, 1 out]
          n99 = call-dynamic "Get Minimum Attenuations.vi"("error in"=w318, "device index (0)"=w309, "rtg api interface"=w315) -> ("error out"=w316:errorcluster, "attenuations (dB)"=w312:dbl[], "rtg api interface out"=w314:refnum<class "NI-RTG Interface.lvclass">)  [unwired: 5 in, 1 out]
          n100 = Array Max & Min(array=w312) -> (max value=w311:dbl, min value=w310:dbl)  [unwired: 2 out]
        }
        "Max Common Attenuations (dB)" <- w303
        "Min Common Attenuations (dB)" <- w304
        "Min Latencies (s)" <- w305
        n101 = Merge Errors(w302) -> (w300:errorcluster)
        n102 = Bundle By Name(cluster=w307, "RTG Ref"=w297) -> (w308:T14)
      }
      frame "RTG_SetPRIs" {
        n103 = Unbundle By Name(w327) -> ("RTG Ref"=w321:refnum<class "NI-RTG Interface.lvclass">)
        n104 = case shown="True" "Set PRIs" {
          tunnel: w321 -> [w329 w331]
          tunnel: [w329 w333] -> w320
          tunnel: w323 -> [w328 w330]
          tunnel: [w328 w332] -> w322
          tunnel: "PRI (s)" -> [_ w334]
          frame False {
          }
          frame True {
            n105 = for {
              tunnel: w334 -> [w340] mode=indexing
              shift-right: [w338] -> w333
              shift-left: w331 -> [w336]
              shift-right: [w337] -> w332
              shift-left: w330 -> [w335]
              i -> [w339]
              n106 = call-dynamic "Set PRI.vi"("error in"=w335, "pri (s)"=w340, "device index (0)"=w339, "NI-RTG Interface in"=w336) -> ("error out"=w337:errorcluster, "NI-RTG Interface out"=w338:refnum<class "NI-RTG Interface.lvclass">)  [unwired: 6 in]
            }
          }
        }
        n107 = Bundle By Name(cluster=w327, "RTG Ref"=w320) -> (w326:T14)
      }
      frame "RTG_CommAtten" {
        # "Begin regularly checking\nCoProcessor"
        # "17"
        n108 = Enqueue Element(queue=w341, element=cluster{"Enum":T12, "Data":variant} {"Enum"=enum."CoPr_Chk", "Data"=variant}, error in (no error)=w342) -> (error out=w343:errorcluster)  [unwired: 1 in, 2 out]
        n109 = Unbundle By Name(w357) -> ("RTG Ref"=w354:refnum<class "NI-RTG Interface.lvclass">, "Index"=w353:i32)
        n110 = call-dynamic "Set Common Attenuation.vi"("error in"=w343, "attenuation (dB)"="Common Attenuation (dB)", "device index (0)"=w353, "rtg api interface"=w354) -> ("error out"=w349:errorcluster, "rtg api interface out"=w352:refnum<class "NI-RTG Interface.lvclass">)  [unwired: 5 in, 1 out]
        n111 = Bundle By Name(cluster=w357, "RTG Ref"=w352) -> (w356:T14)
        n112 = To Variant(anything=Program_Status_Enum."RTG Inactive" ("Status")) -> (Variant=w346:variant)
        n113 = Bundle By Name(cluster=cluster{"Enum":T16, "Var":variant} {"Enum"=enum."Spvsr_UpdtFP", "Var"=variant}, "Var"=w346) -> (w350:cluster{"Enum":T16, "Var":variant})
        n114 = Enqueue Element(queue=w345, element=w350, error in (no error)=w349) -> (error out=w348:errorcluster)  [unwired: 1 in, 2 out]
      }
      frame "RTG_Start" {
        # "Starts the RTG running on the VST."
        n115 = Unbundle By Name(w365) -> ("RTG Ref"=w368:refnum<class "NI-RTG Interface.lvclass">)
        n116 = call-dynamic "Start.vi"("error in"=w369, "rtg api interface"=w368) -> ("error out"=w360:errorcluster, "rtg api interface out"=w367:refnum<class "NI-RTG Interface.lvclass">)  [unwired: 8 in]
        n117 = Bundle By Name(cluster=w365, "RTG Ref"=w367) -> (w366:T14)
        n118 = To Variant(anything=Program_Status_Enum."RTG active" ("Status")) -> (Variant=w361:variant)
        n119 = Bundle By Name(cluster=cluster{"Enum":T16, "Var":variant} {"Enum"=enum."Spvsr_UpdtFP", "Var"=variant}, "Var"=w361) -> (w363:cluster{"Enum":T16, "Var":variant})
        n120 = Enqueue Element(queue=w358, element=w363, error in (no error)=w360) -> (error out=w359:errorcluster)  [unwired: 1 in, 2 out]
      }
      frame "RTG_Stop" {
        # "The Stop is also used to end any current file transfer or target motion operation in progress."
        n121 = local write "Stop RTG"(FALSE ("Stop RTG")) -> ()
        n122 = Unbundle By Name(w381) -> ("RTG Ref"=w380:refnum<class "NI-RTG Interface.lvclass">)
        n123 = call-dynamic "Stop.vi"("error in"=w378, "rtg api interface"=w380) -> ("error out"=w372:errorcluster, "rtg api interface out"=w379:refnum<class "NI-RTG Interface.lvclass">)  [unwired: 8 in]
        n124 = Bundle By Name(cluster=w381, "RTG Ref"=w379) -> (w382:T14)
        n125 = To Variant(anything=Program_Status_Enum."RTG Inactive" ("Status")) -> (Variant=w373:variant)
        n126 = Bundle By Name(cluster=cluster{"Enum":T16, "Var":variant} {"Enum"=enum."Spvsr_UpdtFP", "Var"=variant}, "Var"=w373) -> (w375:cluster{"Enum":T16, "Var":variant})
        n127 = Enqueue Element(queue=w370, element=w375, error in (no error)=w372) -> (error out=w371:errorcluster)  [unwired: 1 in, 2 out]
      }
      frame "RTG_TargetSetup" {
        n128 = Bundle By Name(cluster=w386, "Index"="Device Index", "AutoSend"="Auto Send Software Trigger", "Prepend"="Prepend Software Trigger") -> (w387:T14)
      }
      frame "RTG_Send Target Cfg" {
        # "21"
        n129 = Unbundle By Name(w392) -> ("RTG Ref"=w393:refnum<class "NI-RTG Interface.lvclass">, "Index"=w389:i32)
        n130 = call-dynamic "Send Target Configuration.vi"("error in"=w395, "target config"="Target Configuration", "device index (0)"=w389, "rtg api interface"=w393) -> ("error out"=w394:errorcluster, "rtg api interface out"=w390:refnum<class "NI-RTG Interface.lvclass">)  [unwired: 5 in, 1 out]
        n131 = Bundle By Name(cluster=w392, "RTG Ref"=w390) -> (w391:T14)
      }
      frame "RTG_Send Files" {
        # "----------------------------------20----------------------------------"
        # "21"
        n132 = Unbundle By Name(w410) -> ("AutoSend"=w398:bool, "Prepend"=w397:bool, "RTG Ref"=w399:refnum<class "NI-RTG Interface.lvclass">, "Index"=w400:i32)
        n133 = case shown="True" w397 {
          tunnel: w399 -> [w419 w424]
          tunnel: w403 -> [w418 w421]
          tunnel: w400 -> [_ w423]
          tunnel: [w419 w422] -> w404
          tunnel: [w418 w420] -> w408
          frame False {
          }
          frame True {
            # "requires software trigger"
            n134 = call-dynamic "Send Target Configuration.vi"("error in"=w421, "target config"=T3 {"synchronization"={"synch mode"=enum."Software Trigger", "time offset (s)"=0.0}, "rtg targets"=[{"time offset (s)"=0.0, "attenuaton (dB)"=0.0, "doppler"=0.0, "target enable"=FALSE, "relative velocity enable"=FALSE}, {"time offset (s)"=0.0, "attenuaton (dB)"=0.0, "doppler"=0.0, "target enable"=FALSE, "relative velocity enable"=FALSE}, {"time offset (s)"=0.0, "attenuaton (dB)"=0.0, "doppler"=0.0, "target enable"=FALSE, "relative velocity enable"=FALSE}, {"time offset (s)"=0.0, "attenuaton (dB)"=0.0, "doppler"=0.0, "target enable"=FALSE, "relative velocity enable"=FALSE}]}, "device index (0)"=w423, "rtg api interface"=w424) -> ("error out"=w420:errorcluster, "rtg api interface out"=w422:refnum<class "NI-RTG Interface.lvclass">)  [unwired: 5 in, 1 out]
          }
        }
        n135 = call-dynamic "Send Target Configuration List - Files.vi"("error in"=w408, "target configuration file path"="Target Configuration Files", "device index (0)"=w400, "rtg api interface"=w404) -> ("error out"=w407:errorcluster, "rtg api interface out"=w406:refnum<class "NI-RTG Interface.lvclass">)  [unwired: 6 in]
        n136 = case shown="True" w398 {
          tunnel: w406 -> [w412 w417]
          tunnel: [w412 w416] -> w401
          tunnel: w407 -> [w411 w415]
          tunnel: [w411 w414] -> w402
          tunnel: w400 -> [_ w413]
          frame False {
          }
          frame True {
            n137 = call-dynamic "Send Software Trigger.vi"("error in"=w415, "device index (0)"=w413, "NI-RTG Interface in"=w417) -> ("error out"=w414:errorcluster, "NI-RTG Interface out"=w416:refnum<class "NI-RTG Interface.lvclass">)  [unwired: 7 in]
          }
        }
        n138 = Bundle By Name(cluster=w410, "RTG Ref"=w401) -> (w409:T14)
      }
      frame "RTG_Send Motion" {
        # "----------------------------22----------------------------"
        n139 = Unbundle By Name(w439) -> ("AutoSend"=w426:bool, "Prepend"=w427:bool, "RTG Ref"=w429:refnum<class "NI-RTG Interface.lvclass">, "Index"=w428:i32)
        n140 = case shown="True" w427 {
          tunnel: w429 -> [w448 w453]
          tunnel: w432 -> [w447 w450]
          tunnel: w428 -> [_ w452]
          tunnel: [w448 w451] -> w433
          tunnel: [w447 w449] -> w437
          frame False {
          }
          frame True {
            # "requires software trigger"
            n141 = call-dynamic "Send Target Configuration.vi"("error in"=w450, "target config"=T3 {"synchronization"={"synch mode"=enum."Software Trigger", "time offset (s)"=0.0}, "rtg targets"=[{"time offset (s)"=0.0, "attenuaton (dB)"=0.0, "doppler"=0.0, "target enable"=FALSE, "relative velocity enable"=FALSE}, {"time offset (s)"=0.0, "attenuaton (dB)"=0.0, "doppler"=0.0, "target enable"=FALSE, "relative velocity enable"=FALSE}, {"time offset (s)"=0.0, "attenuaton (dB)"=0.0, "doppler"=0.0, "target enable"=FALSE, "relative velocity enable"=FALSE}, {"time offset (s)"=0.0, "attenuaton (dB)"=0.0, "doppler"=0.0, "target enable"=FALSE, "relative velocity enable"=FALSE}]}, "device index (0)"=w452, "rtg api interface"=w453) -> ("error out"=w449:errorcluster, "rtg api interface out"=w451:refnum<class "NI-RTG Interface.lvclass">)  [unwired: 5 in, 1 out]
          }
        }
        n142 = call-dynamic "Send Target Configuration List - Target Motion.vi"("error in"=w437, "target motion parameters"="Target Motion Parameters", "device index (0)"=w428, "rtg api interface"=w433) -> ("error out"=w435:errorcluster, "rtg api interface out"=w434:refnum<class "NI-RTG Interface.lvclass">)  [unwired: 6 in]
        n143 = case shown="True" w426 {
          tunnel: w434 -> [w441 w446]
          tunnel: [w441 w445] -> w430
          tunnel: w435 -> [w440 w444]
          tunnel: [w440 w443] -> w431
          tunnel: w428 -> [_ w442]
          frame False {
          }
          frame True {
            n144 = call-dynamic "Send Software Trigger.vi"("error in"=w444, "device index (0)"=w442, "NI-RTG Interface in"=w446) -> ("error out"=w443:errorcluster, "NI-RTG Interface out"=w445:refnum<class "NI-RTG Interface.lvclass">)  [unwired: 7 in]
          }
        }
        n145 = Bundle By Name(cluster=w439, "RTG Ref"=w430) -> (w438:T14)
      }
      frame "RTG_Send SW Trigg" {
        n146 = Unbundle By Name(w461) -> ("RTG Ref"=w456:refnum<class "NI-RTG Interface.lvclass">, "Index"=w457:i32)
        n147 = call-dynamic "Send Software Trigger.vi"("error in"=w459, "device index (0)"=w457, "NI-RTG Interface in"=w456) -> ("error out"=w458:errorcluster, "NI-RTG Interface out"=w455:refnum<class "NI-RTG Interface.lvclass">)  [unwired: 7 in]
        n148 = Bundle By Name(cluster=w461, "RTG Ref"=w455) -> (w460:T14)
      }
      frame "RTG_Chk" {
        n149 = Wait Until Next ms Multiple(millisecond multiple=u32 100) -> ()  [unwired: 1 out]
        n150 = Enqueue Element(queue=w470, element=cluster{"Enum":T15, "Var":variant} {"Enum"=enum."RTG_Chk", "Var"=variant}, error in (no error)=w471) -> (error out=w472:errorcluster)  [unwired: 1 in, 2 out]
        n151 = Unbundle By Name(w476) -> ("RTG Ref"=w473:refnum<class "NI-RTG Interface.lvclass">)
        n152 = call-dynamic "Get Coprocessor Link Status.vi"("error in"=w472, "rtg api interface"=w473) -> ("error out"=w466:errorcluster, "rtg link status"=→"rtg link status":T9[], "rtg api interface out"=w464:refnum<class "NI-RTG Interface.lvclass">)  [unwired: 7 in]
        n153 = call-dynamic "Get RTG Status.vi"("error in"=w466, "rtg api interface"=w464) -> ("error out"=w465:errorcluster, "rtg status"=→"RTG Status":string, "state"=w462:T10, "rtg api interface out"=w463:refnum<class "NI-RTG Interface.lvclass">)  [unwired: 6 in]
        "RTG State" <- w462
        n154 = Bundle By Name(cluster=w476, "RTG Ref"=w463, "state"=w462) -> (w475:T14)
      }
      frame "RTG_Exit" {
        # "RTG Exit is called from Coprocesor Exit\nto prevent a race condition"
        n155 = Unbundle By Name(w478) -> ("RTG Ref"=w479:refnum<class "NI-RTG Interface.lvclass">)
        n156 = call-dynamic "Close.vi"("error in"=w481, "rtg api interface"=w479) -> ("error out"=w482:errorcluster, "rtg api interface out"=w483:refnum<class "NI-RTG Interface.lvclass">)  [unwired: 8 in]
        n157 = call-dynamic "Destroy.vi"("error in"=w482, "NI-RTG Interface in"=w483) -> ("error out"=w480:errorcluster)  [unwired: 9 in]
      }
    }
    n158 = call "Log_Errors_20190313.vi"("LoopName"="RTG", "error in"=w146) -> ("error out"=w145:errorcluster)  [unwired: 9 in]
  }
  n159 = while {
    tunnel: w20 -> [w486]
    tunnel: w1 -> [w484]
    stop <- w485 stop-if-true
    # "Event Loop"
    n160 = event shown="[2] \"Commit HW\": Value Change" {
      selector: _ -> [_ _ _ _ _ _ _ _ _ _]
      dyn-events: _ -> [_ _ _ _ _ _ _ _ _ _]
      timeout: 200 -> [_ _ _ _ _ _ _ _ _ _]
      tunnel: w486 -> [_ _ w493 _ _ _ _ _ _ w522]
      tunnel: [_ _ _ _ _ _ _ _ _ TRUE] -> w485
      tunnel: w484 -> [_ w490 _ w498 w502 w506 w510 w514 w518 _]
      event Timeout {
        n161 = event-data() -> ()  [unwired: 1 in, 3 out]
        n162 = Get Date/Time String() -> (time string=→"System Time":string)  [unwired: 3 in, 1 out]
      }
      event "Start RTG": Value Change {
        n163 = event-data() -> ()  [unwired: 1 in, 6 out]
        n164 = Enqueue Element(queue=w490, element=cluster{"Enum":T15, "Var":variant} {"Enum"=enum."RTG_Start", "Var"=variant}) -> (error out=w491:errorcluster)  [unwired: 2 in, 2 out]
        n165 = call "Log_Errors_20190313.vi"("LoopName"="EventStart", "error in"=w491) -> ()  [unwired: 9 in, 1 out]
      }
      event "Commit HW": Value Change {
        n166 = event-data() -> ()  [unwired: 1 in, 6 out]
        n167 = Enqueue Element(queue=w493, element=cluster{"Enum":T16, "Var":variant} {"Enum"=enum."Spvsr_InitRTG", "Var"=variant}) -> (error out=w495:errorcluster)  [unwired: 2 in, 2 out]
        n168 = call "Log_Errors_20190313.vi"("LoopName"="EventStart", "error in"=w495) -> ()  [unwired: 9 in, 1 out]
      }
      event "Send SW Trigg": Value Change {
        n169 = event-data() -> ()  [unwired: 1 in, 6 out]
        n170 = Enqueue Element(queue=w498, element=cluster{"Enum":T15, "Var":variant} {"Enum"=enum."RTG_Send SW Trigg", "Var"=variant}) -> (error out=w499:errorcluster)  [unwired: 2 in, 2 out]
        n171 = call "Log_Errors_20190313.vi"("LoopName"="SW_Trigg", "error in"=w499) -> ()  [unwired: 9 in, 1 out]
      }
      event "Stop RTG": Value Change {
        n172 = event-data() -> ()  [unwired: 1 in, 6 out]
        n173 = Enqueue Element(queue=w502, element=cluster{"Enum":T15, "Var":variant} {"Enum"=enum."RTG_Stop", "Var"=variant}) -> (error out=w503:errorcluster)  [unwired: 2 in, 2 out]
        n174 = call "Log_Errors_20190313.vi"("LoopName"="EventStop", "error in"=w503) -> ()  [unwired: 9 in, 1 out]
      }
      event "Device Index", "Prepend Software Trigger", "Auto Send Software Trigger": Value Change {
        n175 = event-data() -> ()  [unwired: 1 in, 6 out]
        n176 = Enqueue Element(queue=w506, element=cluster{"Enum":T15, "Var":variant} {"Enum"=enum."RTG_TargetSetup", "Var"=variant}) -> (error out=w507:errorcluster)  [unwired: 2 in, 2 out]
        n177 = call "Log_Errors_20190313.vi"("LoopName"="DevIndex", "error in"=w507) -> ()  [unwired: 9 in, 1 out]
      }
      event "Send TrgtCfg": Value Change {
        n178 = event-data() -> ()  [unwired: 1 in, 6 out]
        n179 = Enqueue Element(queue=w510, element=cluster{"Enum":T15, "Var":variant} {"Enum"=enum."RTG_Send Target Cfg", "Var"=variant}) -> (error out=w511:errorcluster)  [unwired: 2 in, 2 out]
        n180 = call "Log_Errors_20190313.vi"("LoopName"="SendTargetCfg", "error in"=w511) -> ()  [unwired: 9 in, 1 out]
      }
      event "Send Motion": Value Change {
        n181 = event-data() -> ()  [unwired: 1 in, 6 out]
        n182 = Enqueue Element(queue=w514, element=cluster{"Enum":T15, "Var":variant} {"Enum"=enum."RTG_Send Motion", "Var"=variant}) -> (error out=w515:errorcluster)  [unwired: 2 in, 2 out]
        n183 = call "Log_Errors_20190313.vi"("LoopName"="SendMotion", "error in"=w515) -> ()  [unwired: 9 in, 1 out]
      }
      event "Send Files": Value Change {
        n184 = event-data() -> ()  [unwired: 1 in, 6 out]
        n185 = Enqueue Element(queue=w518, element=cluster{"Enum":T15, "Var":variant} {"Enum"=enum."RTG_Send Files", "Var"=variant}) -> (error out=w519:errorcluster)  [unwired: 2 in, 2 out]
        n186 = call "Log_Errors_20190313.vi"("LoopName"="SendFiles", "error in"=w519) -> ()  [unwired: 9 in, 1 out]
      }
      event "Exit": Value Change {
        n187 = event-data() -> ()  [unwired: 1 in, 6 out]
        n188 = To Variant(anything=Program_Status_Enum."Closing" ("Status")) -> (Variant=w523:variant)
        n189 = Bundle By Name(cluster=cluster{"Enum":T16, "Var":variant} {"Enum"=enum."Spvsr_UpdtFP", "Var"=variant}, "Var"=w523) -> (w525:cluster{"Enum":T16, "Var":variant})
        n190 = Enqueue Element(queue=w522, element=w525) -> (queue out=w521:refnum<queue>)  [unwired: 2 in, 2 out]
        n191 = Enqueue Element(queue=w521, element=cluster{"Enum":T16, "Var":variant} {"Enum"=enum."Spvsr_Exit", "Var"=variant}) -> (error out=w528:errorcluster)  [unwired: 2 in, 2 out]
        n192 = call "Log_Errors_20190313.vi"("LoopName"="EventExit", "error in"=w528) -> ()  [unwired: 9 in, 1 out]
      }
    }
  }
  n193 = while {
    tunnel: w12 -> [w542]
    tunnel: [w544] -> w4
    tunnel: w2 -> [w541]
    tunnel: w1 -> [w538]
    tunnel: w20 -> [w531]
    shift-right: [w537] -> _
    shift-left: T13 {"CoPr Refs"=[]} -> [w536]
    stop <- w532 stop-if-true
    # "CoProcessor Loop"
    n194 = Dequeue Element(queue=w541, error in (no error)=w542) -> (queue out=w533:refnum<queue>, element=w543:cluster{"Enum":T12, "Data":variant}, error out=w535:errorcluster)  [unwired: 1 in, 1 out]
    n195 = Unbundle(w543) -> ("Enum"=w540:T12, "Data"=w539:variant)
    n196 = case shown="\"CoPr_Chk\"" w540 {
      tunnel: w539 -> [w559 _ _]
      tunnel: w538 -> [w554 _ w616]
      tunnel: [w563 w579 w619] -> w537
      tunnel: w536 -> [w562 w579 w619]
      tunnel: w535 -> [w560 w588 w614]
      tunnel: [w555 w577 w621] -> w534
      tunnel: w533 -> [_ w587 _]
      tunnel: [_ _ TRUE] -> w532
      tunnel: w531 -> [_ w576 _]
      frame "CoPr_Init" {
        # "3. Create and Intialize Coprocessor Object if valid Coprocessor Hardware"
        # "3"
        n197 = Variant To Data(error in=w560, type="" ("option string"), Variant=w559) -> (data=w557:string, error out=w561:errorcluster)
        n198 = call <vilib>:"Create Coprocessor.vi"("error in"=w561, "option string"=w557, "coprocessor resources"="Coprocessor Names") -> ("error out"=w556:errorcluster, "rtg coprocessor links"=w551:refnum<class "RTG Coprocessor Link Interface.lvclass">[])  [unwired: 7 in]
        n199 = Bundle By Name(cluster=w562, "CoPr Refs"=w551) -> (w563:T13)
        n200 = To Variant(anything=w551) -> (Variant=w550:variant)
        n201 = Bundle By Name(cluster=cluster{"Enum":T15, "Var":variant} {"Enum"=enum."RTG_RefLvl", "Var"=variant}, "Var"=w550) -> (w552:cluster{"Enum":T15, "Var":variant})
        n202 = Build Array(w552, cluster{"Enum":T15, "Var":variant} {"Enum"=enum."RTG_mmWav", "Var"=variant}, cluster{"Enum":T15, "Var":variant} {"Enum"=enum."RTG_Cal", "Var"=variant}, cluster{"Enum":T15, "Var":variant} {"Enum"=enum."RTG_CalDone?", "Var"=variant}) -> (w549:cluster{"Enum":T15, "Var":variant}[])
        n203 = for {
          tunnel: w554 -> [w566]
          tunnel: w549 -> [w565] mode=indexing
          shift-right: [w567] -> w555
          shift-left: w556 -> [w568]
          n204 = Enqueue Element(queue=w566, element=w565, error in (no error)=w568) -> (error out=w567:errorcluster)  [unwired: 1 in, 2 out]
        }
      }
      frame "CoPr_Chk" {
        # "Send count\nwhen it \nchanges"
        n205 = Unbundle By Name(w579) -> ("CoPr Refs"=w580:refnum<class "RTG Coprocessor Link Interface.lvclass">[])
        n206 = Wait Until Next ms Multiple(millisecond multiple=u32 100) -> ()  [unwired: 1 out]
        n207 = Enqueue Element(queue=w587, element=cluster{"Enum":T12, "Data":variant} {"Enum"=enum."CoPr_Chk", "Data"=variant}, error in (no error)=w588) -> (error out=w581:errorcluster)  [unwired: 1 in, 2 out]
        n208 = for {
          tunnel: w580 -> [w601] mode=indexing
          tunnel: [w605] -> w582 mode=indexing
          shift-right: [w598] -> w578
          shift-left: w581 -> [w606]
          tunnel: [w600] -> w584 mode=indexing
          tunnel: [w594] -> w583 mode=indexing
          n209 = call-dynamic "Get Coprocessor Refnum.vi"("rtg coprocessor link interface"=w601) -> ("error out"=w604:errorcluster, "coprocessor refnum"=w602:refnum<k20>)  [unwired: 8 in, 1 out]
          n210 = call-dynamic "Coprocessor Link Status.vi"("error in"=w606, "rtg coprocessor link interface"=w601) -> ("error out"=w596:errorcluster, "coprocessor status out"=w605:T11, "rtg coprocessor link interface out"=w597:refnum<class "RTG Coprocessor Link Interface.lvclass">)  [unwired: 7 in]
          n211 = Not A Number/Path/Refnum?(number/path/refnum=w602) -> (NaN/Path/Refnum?=w603:bool)
          n212 = case shown="False" w603 {
            tunnel: w602 -> [w610 _]
            tunnel: w604 -> [w609 w613]
            tunnel: [w608 w613] -> w599
            tunnel: [w607 _] -> w600
            frame False {
              # "Read RTG coprocessor \nrecieved trigger count"
              n213 = Dynamic FPGA Interface Cast(Session In=refnum<k20> refnum ("Type"), Type=w610) -> (Session Out=w612:refnum<k20>)
              n214 = xnode "Read/Write Control"("FPGA VI Reference In"=w612, "error in"=w609) -> ("error out"=w608:errorcluster, "read trigger rising edge count"=w607:u16)  [unwired: 1 out]
            }
            frame True {
            }
          }
          n215 = call-dynamic "Get Device Index.vi"("error in"=w596, "rtg coprocessor link interface"=w597) -> ("error out"=w595:errorcluster, "device index"=w594:i32)  [unwired: 7 in, 1 out]
          n216 = Merge Errors(w595, w599) -> (w598:errorcluster)
        }
        "coproc link" <- w582
        n217 = Build Array(w583, w584) -> (w570:i32[][])
        n218 = feedback-in #1(w570) -> ()
        n219 = feedback #1(i32[][] []) -> (w571:i32[][])
        n220 = To Variant(anything=w570) -> (Variant=w573:variant)
        n221 = Not Equal?(x=w570, y=w571) -> (x != y?=w569:bool)
        n222 = Bundle By Name(cluster=cluster{"Enum":T16, "Var":variant} {"Enum"=enum."Spvsr_StateCount", "Var"=variant}, "Var"=w573) -> (w574:cluster{"Enum":T16, "Var":variant})
        n223 = case shown="True" w569 {
          tunnel: w578 -> [w589 w593]
          tunnel: [w589 w592] -> w577
          tunnel: w576 -> [_ w591]
          tunnel: w574 -> [_ w590]
          frame False {
          }
          frame True {
            n224 = Enqueue Element(queue=w591, element=w590, error in (no error)=w593) -> (error out=w592:errorcluster)  [unwired: 1 in, 2 out]
          }
        }
      }
      frame "CoPr_Exit" {
        n225 = Enqueue Element(queue=w616, element=cluster{"Enum":T15, "Var":variant} {"Enum"=enum."RTG_Exit", "Var"=variant}, error in (no error)=w614) -> (error out=w615:errorcluster)  [unwired: 1 in, 2 out]
        n226 = Unbundle By Name(w619) -> ("CoPr Refs"=w620:refnum<class "RTG Coprocessor Link Interface.lvclass">[])
        n227 = for {
          tunnel: w620 -> [w624] mode=indexing
          shift-right: [w622] -> w621
          shift-left: w615 -> [w623]
          # "29"
          n228 = call-dynamic "Close.vi"("error in"=w623, "rtg coprocessor link interface"=w624) -> ("error out"=w622:errorcluster)  [unwired: 9 in]
        }
      }
    }
    n229 = call "Log_Errors_20190313.vi"("LoopName"="CoPr", "error in"=w534) -> ("error out"=w544:errorcluster)  [unwired: 9 in]
  }
  n230 = flat-sequence {
    tunnel: w20 -> [w636]
    tunnel: w6 -> [w635]
    tunnel: w5 -> [w634]
    tunnel: w4 -> [w633]
    tunnel: w2 -> [w631]
    tunnel: w1 -> [w630]
    frame #0 {
      w629 = FALSE ("Stop RTG")
      n231 = Release Queue(queue=w636) -> (error out=w626:errorcluster)  [unwired: 2 in, 2 out]
      n232 = Release Queue(queue=w630) -> (error out=w627:errorcluster)  [unwired: 2 in, 2 out]
      n233 = Release Queue(queue=w631) -> (error out=w628:errorcluster)  [unwired: 2 in, 2 out]
      n234 = Merge Errors(w626, w627, w628, w635, w634, w633) -> (w632:errorcluster)
      n235 = local write "error out"(w632) -> ()
      n236 = local write "App Status"(Program_Status_Enum."Closed" ("App Status")) -> ()
      n237 = local write "Stop RTG"(w629) -> ()
      n238 = local write "Exit"(w629) -> ()
    }
  }
